vi "Resolve Service.vi"(8 "error in":errorcluster, 11 "request data":T1) -> (0 "error out":errorcluster, 3 "response data":T2)   [LabVIEW 2020, in "MeasurementLink Discovery.lvlib"]
uses:
  MeasurementLink Discovery.lvlib
  MeasurementLink Discovery Client/RPC Messages/ni_measurementlink_discovery_v1_ServiceLocation.ctl
  MeasurementLink Discovery Client/RPC Messages/ni_measurementlink_discovery_v1_ResolveServiceRequest.ctl
  TypeDefs/gRPC Client Cache FGV Action.ctl
  MeasurementLink Discovery Client/MeasurementLink Discovery Client.lvlib
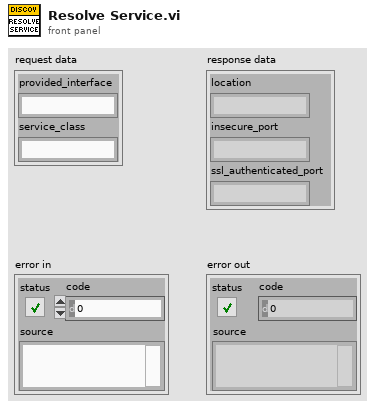
[diagram p1: front panel]
types:
  T1 = typedef "MeasurementLink Discovery Client.lvlib/ni_measurementlink_discovery_v1_ResolveServiceRequest.ctl" = cluster{"provided_interface":string, "service_class":string}
  T2 = typedef "MeasurementLink Discovery Client.lvlib/ni_measurementlink_discovery_v1_ServiceLocation.ctl" = cluster{"location":string, "insecure_port":string, "ssl_authenticated_port":string}
  T3 = typedef "MeasurementLink Discovery.lvlib/gRPC Client Cache FGV Action.ctl" = enum16{"Get Client", "Recreate Client"}
  T4 = typedef "grpc-lvsupport-release.lvlib/grpcId.ctl" = u64
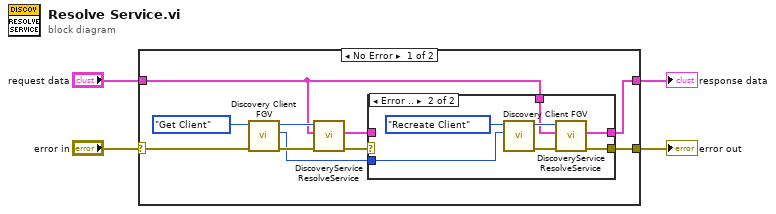
[diagram p0: block diagram]
diagram:
  n1 = case shown="No Error" "error in" {
    selector: "error in" -> [w14 w24]
    tunnel: [w9 w24] -> w3
    tunnel: [w8 _] -> w2
    tunnel: "request data" -> [w6 _]
    frame No Error {
      n2 = call "Discovery Client FGV.vi"("error in"=w14, "action"=gRPC_Client_Cache_FGV_Action."Get Client") -> ("error out"=w12:errorcluster, "unique id out"=w5:u64, "grpc client id"=w11:T4)  [unwired: 7 in]
      n3 = call "DiscoveryService ResolveService.vi"("error in"=w12, "Request Data"=w6, "gRPC ID"=w11) -> ("error out"=w10:errorcluster, "Response Data"=w7:T2)  [unwired: 6 in, 1 out]
      n4 = case shown="Error .." w10 {
        selector: w10 -> [w16 _]
        tunnel: [w16 w20] -> w9
        tunnel: [w15 w19] -> w8
        tunnel: w7 -> [w15 _]
        tunnel: w6 -> [_ w18]
        tunnel: w5 -> [_ w17]
        frame No Error {
        }
        frame Error {
          n5 = call "Discovery Client FGV.vi"("unique id in"=w17, "action"=gRPC_Client_Cache_FGV_Action."Recreate Client") -> ("error out"=w21:errorcluster, "grpc client id"=w22:T4)  [unwired: 7 in, 1 out]
          n6 = call "DiscoveryService ResolveService.vi"("error in"=w21, "Request Data"=w18, "gRPC ID"=w22) -> ("error out"=w20:errorcluster, "Response Data"=w19:T2)  [unwired: 6 in, 1 out]
        }
      }
    }
    frame Error {
    }
  }
  "error out" <- w3
  "response data" <- w2
